vi "总磷单步调试对话框.vi"() -> ()   [LabVIEW 2016, in "斯坦道总磷.lvlib"]
panel:
  in  "退出":bool
  in  "启动":bool
  in  "总磷氨氮调试":u16[](xcontrol)
  # "总磷单步调试界面"
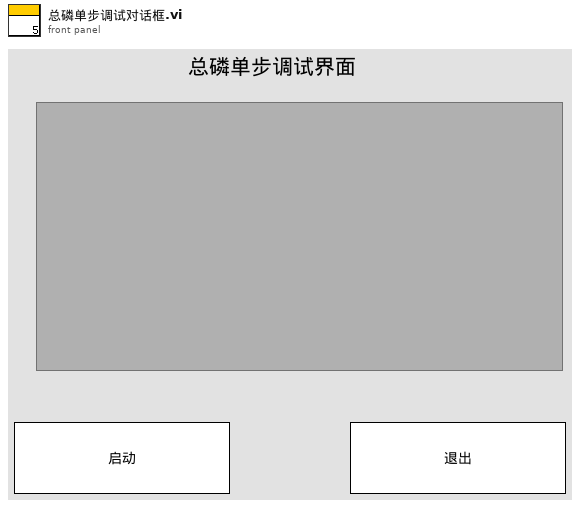
[diagram p1: front panel]
types:
  T1 = cluster{"阀口名称自定义类型":enum16{"自定义", "微站总磷总氮", "微站总磷氨氮", "微站氨氮", "固定站总磷", "固定站总氮", "固定站氨氮", "原位总磷总氮", "原位总磷氨氮", "原位总磷", "原位总氮", "原位氨氮", "原位3N1P"}, "阀口自定义名称":cluster{"V1":string, "V2":string, "V3":string, "V4":string, "V5":string, "V6":string, "V7":string, "V8":string, "V9":string, "V10":string, "V11":string, "V12":string, "V9-1":string, "V9-2":string}}
  T2 = enum16{"自定义", "微站总磷总氮", "微站总磷氨氮", "微站氨氮", "固定站总磷", "固定站总氮", "固定站氨氮", "原位总磷总氮", "原位总磷氨氮", "原位总磷", "原位总氮", "原位氨氮", "原位3N1P"}
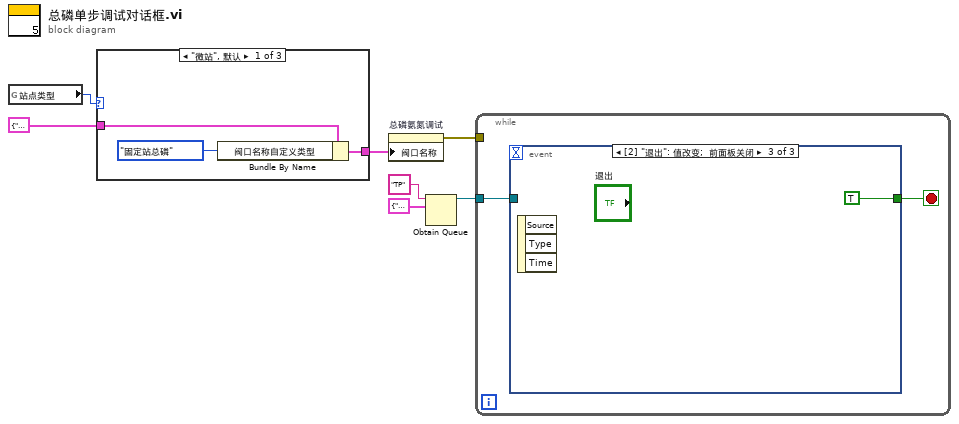
[diagram p0: block diagram]
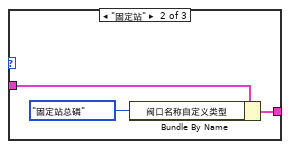
[diagram p2: hidden frame]
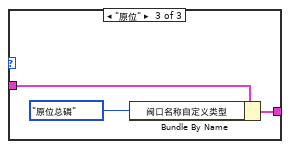
[diagram p3: hidden frame]
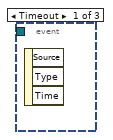
[diagram p4: hidden frame]
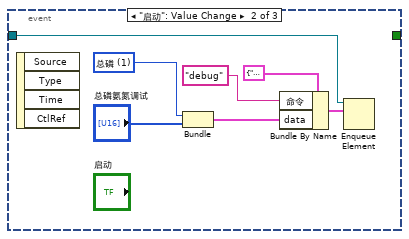
[diagram p5: hidden frame]
diagram:
  n1 = global read "VAR总磷全局变量.vi" "站点类型"() -> (w4:enum16{"微站", "固定站", "原位"})
  n2 = case shown="\"微站\", 默认" w4 {
    tunnel: T1 {"阀口名称自定义类型"=enum."自定义", "阀口自定义名称"={"V1"="", "V2"="", "V3"="", "V4"="", "V5"="", "V6"="", "V7"="", "V8"="", "V9"="", "V10"="", "V11"="", "V12"="", "V9-1"="", "V9-2"=""}} ("阀口名称") -> [w10 w13 w16]
    tunnel: [w9 w12 w15] -> w1
    frame "微站", Default {
      n3 = Bundle By Name(cluster=w10, "阀口名称自定义类型"=T2."固定站总磷") -> (w9:T1)
    }
    frame "固定站" {
      n4 = Bundle By Name(cluster=w13, "阀口名称自定义类型"=T2."固定站总磷") -> (w12:T1)
    }
    frame "原位" {
      n5 = Bundle By Name(cluster=w16, "阀口名称自定义类型"=T2."原位总磷") -> (w15:T1)
    }
  }
  n6 = property on="总磷氨氮调试" class="调试控件V3 (严格)"("阀口名称"=w1) -> (error out=w3:errorcluster)  [unwired: 2 in, 1 out]
  n7 = Obtain Queue(name (unnamed)="TP" ("名称（未命名）"), element data type=cluster{"命令":string, "data":variant} {"命令"="", "data"=variant}) -> (queue out=w5:refnum<queue>)  [unwired: 3 in, 2 out]
  n8 = while {
    tunnel: w5 -> [w18]
    tunnel: w3 -> [_]
    stop <- w17 stop-if-true
    n9 = event shown="[2] \"退出\": 值改变;  前面板关闭" {
      selector: _ -> [_ _ _]
      dyn-events: _ -> [_ _ _]
      timeout: _ -> [_ _ _]
      tunnel: w18 -> [_ w20 _]
      tunnel: [_ _ TRUE] -> w17
      event Timeout {
        n10 = event-data() -> ()  [unwired: 1 in, 3 out]
      }
      event "启动": Value Change {
        w22 = u16 1 items=["总磷"=1, "氨氮"=3] ("站号")
        n11 = event-data() -> ()  [unwired: 1 in, 4 out]
        n12 = Bundle("站号"=w22, "总磷氨氮调试"="总磷氨氮调试") -> (w21:cluster{"站号":u16, "总磷氨氮调试":u16[]})  [unwired: 1 in]
        n13 = Bundle By Name(cluster=cluster{"命令":string, "data":variant} {"命令"="", "data"=variant} ("元素"), "命令"="debug", "data"=w21) -> (w23:cluster{"命令":string, "data":variant})
        n14 = Enqueue Element(queue=w20, element=w23) -> ()  [unwired: 2 in, 3 out]
      }
      event "退出": Value Change; Panel Close {
        n15 = event-data() -> ()  [unwired: 1 in, 3 out]
      }
    }
  }
